vi "SimpleRandom.vi"() -> (1 "nearest integer value":dbl)   [LabVIEW 2013]
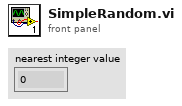
[diagram p1: front panel]
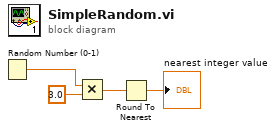
[diagram p0: block diagram]
diagram:
  n1 = Random Number (0-1)() -> (number: 0 to 1=w4:dbl)
  n2 = Multiply(x=w4, y=3.0) -> (x*y=w2:dbl)
  n3 = Round To Nearest(number=w2) -> (nearest integer value=→"nearest integer value":dbl)
